vi "Motic Close Camera.vi"(8 "error in (no error)":errorcluster, 11 "camera":i32) -> (0 "error out":errorcluster, 3 "camera out":i32)   [LabVIEW 2012, in "MoticApi.lvlib"]
doc: "MOTICAPI void Motic_CloseCamera(MUCam_Handle camera);"
uses:
  MoticApi.lvlib
  MoticApi.dll
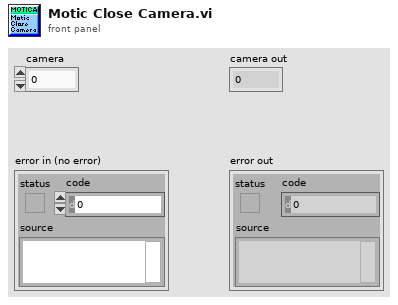
[diagram p1: front panel]
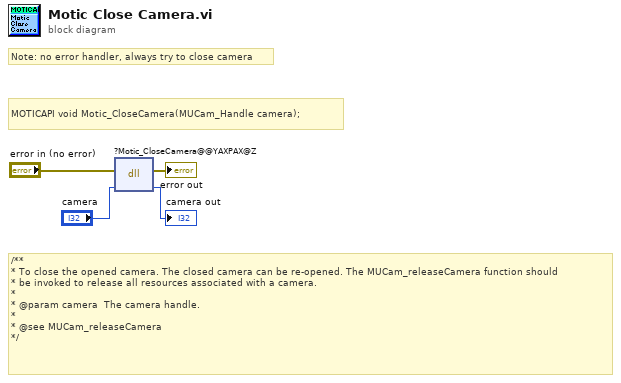
[diagram p0: block diagram]
diagram:
  # "Note: no error handler, always try to close camera"
  # "/**\n* To close the opened camera. The closed camera can be re-opened. The MUCam_releaseCamera function should\n* be invoked to release all resources associated with a camera.\n*\n* @param camera  The camera handle.\n*\n* @see MUCam_releaseCamera\n*/"
  # "MOTICAPI void Motic_CloseCamera(MUCam_Handle camera);"
  n1 = dll-call lib="C:/Users/TTS-Digital/Desktop/MoticApi/MoticApi_git/MoticApi/MoticApi.*" fn="?Motic_CloseCamera@@YAXPAX@Z"(error in="error in (no error)", "camera"="camera") -> (error out=→"error out":errorcluster, "camera"=→"camera out":i32)  [unwired: 3 in, 1 out]
